vi "Convert 2D Array to map.vi"(0 "Map in":map{string, dbl}(c390), 5 "String Array":string[][](array[string])) -> (4 "Map out":map{string, dbl}(c390))   [LabVIEW 2020]
doc: "This VI is used to convert the 2d array of the data into the map. It accepts 2D string array and converts it into the map. The type of the map is \nkey -> String\nValue -> DBL"
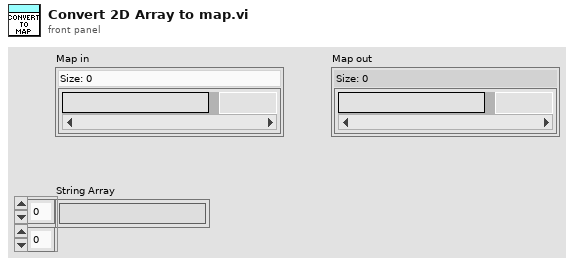
[diagram p1: front panel]
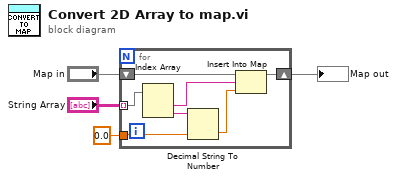
[diagram p0: block diagram]
diagram:
  n1 = for {
    tunnel: "String Array" -> [w11] mode=indexing
    shift-right: [w7] -> w3
    shift-left: "Map in" -> [w6]
    tunnel: 0.0 ("Type Of 2nd Index Numeric") -> [w5]
    n2 = Index Array(array=w11) -> (element #1=w10:string, element #2=w9:string)  [unwired: 2 in]
    n3 = Decimal String To Number(string=w9, default (0L)=w5) -> (number=w8:dbl)  [unwired: 1 in, 1 out]
    n4 = Insert Into Map(map in=w6, key=w10, value=w8) -> (map out=w7:map{string, dbl})  [unwired: 2 out]
  }
  "Map out" <- w3
